vi "Configure Keyboard lock.vi"(8 "error in (no error)":errorcluster, 10 "Lock Keyboard (F: Unlock)":bool, 11 "VISA resource name":refnum<visa-resource-name>) -> (0 "error out":errorcluster, 3 "VISA resource name out":refnum<visa-resource-name>)   [LabVIEW 2017, in "RadWag balances and scales.lvlib"]
doc: "Locks or unlocks the keyboard.\nWhen the keyboard is locked, no configuration changes can be applied from balance front panel."
uses:
  <instrlib>/Radwag Balances and Scales/Public/RadWag balances and scales.lvlib
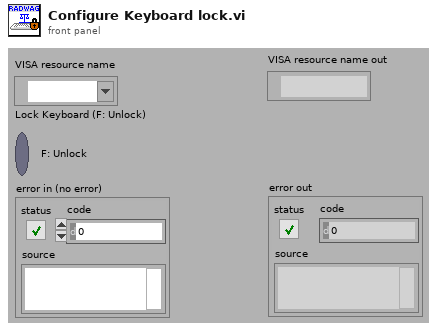
[diagram p1: front panel]
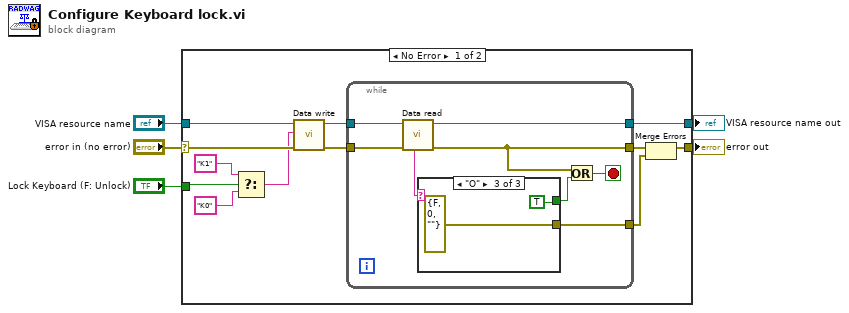
[diagram p0: block diagram]
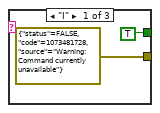
[diagram p2: hidden frame]
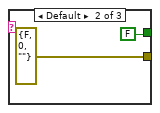
[diagram p3: hidden frame]
diagram:
  n1 = case shown="No Error" "error in (no error)" {
    selector: "error in (no error)" -> [w13 w32]
    tunnel: "Lock Keyboard (F: Unlock)" -> [w10 _]
    tunnel: "VISA resource name" -> [w17 w33]
    tunnel: [w15 w33] -> w3
    tunnel: [w7 w32] -> w2
    frame No Error {
      n2 = Select(t="K1", s=w10, f="K0") -> (s? t:f=w9:string)
      n3 = call <instrlib>:"Data write.vi"("error in (no error)"=w13, "ID"=w9, "VISA resource name"=w17) -> ("error out"=w14:errorcluster, "VISA resource name out"=w16:refnum<visa-resource-name>)  [unwired: 7 in]
      n4 = while {
        tunnel: w16 -> [w25]
        tunnel: [w24] -> w15
        tunnel: w14 -> [w23]
        tunnel: [w21] -> w8
        tunnel: [w18] -> w6
        stop <- w22 stop-if-true
        n5 = call <instrlib>:"Data read.vi"("error in (no error)"=w23, "VISA resource name"=w25) -> ("error out"=w21:errorcluster, "VISA resource name out"=w24:refnum<visa-resource-name>, "Status"=w20:string)  [unwired: 3 in, 4 out]
        n6 = case shown="\"O\"" w20 {
          tunnel: [errorcluster {"status"=FALSE, "code"=1073481728, "source"="Warning: Command currently unavailable"} ("t") errorcluster {"status"=FALSE, "code"=0, "source"=""} ("error constant") errorcluster {"status"=FALSE, "code"=0, "source"=""} ("error constant")] -> w18
          tunnel: [TRUE FALSE TRUE] -> w19
          frame "I" {
          }
          frame Default {
          }
          frame "O" {
          }
        }
        n7 = Or(x=w21, y=w19) -> (x .or. y?=w22:bool)
      }
      n8 = Merge Errors(w8, w6) -> (w7:errorcluster)
    }
    frame Error {
    }
  }
  "VISA resource name out" <- w3
  "error out" <- w2
